vi "Test Find Extrema.vi"() -> ()   [LabVIEW 2013]
uses:
  Empirical Mode Decomposition.lvlib
panel:
  in  "peaks/valleys":enum32{"Peaks", "Valleys"}(ring)=enum."Valleys"
  out "# Zero Crossings":i32
  out "Amplitudes":dbl[](array[numeric])
  out "Indicies":u32[](array[numeric])
  in  "Array":dbl[](array[numeric])
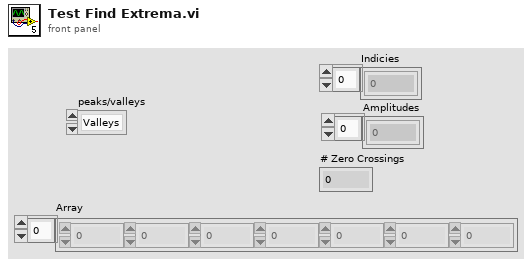
[diagram p1: front panel]
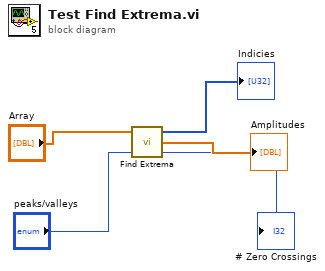
[diagram p0: block diagram]
diagram:
  n1 = call "Find Extrema.vi"("peaks/valleys"="peaks/valleys", "Array"="Array") -> ("# Zero Crossings"=→"# Zero Crossings":i32, "Amplitudes"=→"Amplitudes":dbl[], "Indicies"=→"Indicies":u32[])  [unwired: 1 in]
